vi "Main.vi"(11 "Module Admin":refnum<class "Delacor_lib_QMH_Module Admin.lvclass">) -> ()   [LabVIEW 2019, in "ContextHelp.lvlib"]
doc: "This template is based off of the Queued Message Handler design pattern and the Queued Message Handler project template that ships with LabVIEW.\n\nThe main difference is that the queue is private to this module and communication between modules is performed via Broadcast and Request events.\n\nRequest events are wrapped in public API methods and are handled in the Event Handling Loop (EHL) of this VI. Any module can register for Broadcast events sent by this module. The EHL generates messages based on user interface actions.\n\nThe Message Handling Loop (MHL) processes messages generated by the EHL, or by other messages. The messages are string values, so new messages can be added easily to the Message Cases case structure in the MHL. Each message cluster can also provide an optional value for Message Data, which is a variant that can be converted to whatever message-specific data is required.\n_____\nBased on DQMH Project Template 6.1.0.94.\n____\nPantherLAB Templates 1.0.0.5\nCopyright (c) 2022, PantherLAB"
uses:
  ContextHelp.lvlib
  <vilib>/Delacor/Delacor QMH/Libraries/Module Admin_class/Delacor_lib_QMH_Module Admin.lvclass
  Module Data--cluster.ctl
  <vilib>/Delacor/Delacor QMH/Libraries/Message Queue_class/Delacor_lib_QMH_Message Queue.lvclass/Delacor_lib_QMH_Message Queue.ctl
  Stop Argument--cluster.ctl
  <vilib>/Delacor/Delacor QMH/Libraries/Module Admin_class/Delacor_lib_QMH_Module Admin.lvclass/Delacor_lib_QMH_Module Admin.ctl
  Draw Panel Into Subpanel Argument--cluster.ctl
  Remove Panel from Subpanel Argument--cluster.ctl
  <vilib>/Delacor/Delacor QMH/Libraries/Message Queue_class/Delacor_lib_QMH_Enqueue Message (Single).vi
  <vilib>/Delacor/Delacor QMH/Libraries/Module Admin_class/Delacor_lib_QMH_Get External Launch.vi
  <vilib>/Utility/error.llb/Error Cluster From Error Code.vi
  <vilib>/ErrorRing/Error Ring.xnode
  <vilib>/Delacor/Delacor QMH/Libraries/Message Queue_class/Delacor_lib_QMH_Message Queue.lvclass
  Panther Dashboard/Panther Dashboard.lvlib
  Shared/Shared.lvlib
panel:
  out "Status":string
  out "error out":errorcluster
  in  "Edit Project Description":bool caption="Project Documentation"
  in  "Project Description":string
  in  "Edit Module Description":bool caption="Module Description"
  in  "Module Description":string
  in  "Edit VI":bool caption="Event Connector Pane- Edit"
  out "Event Connector Pane":picture
  in  "Event Description":string
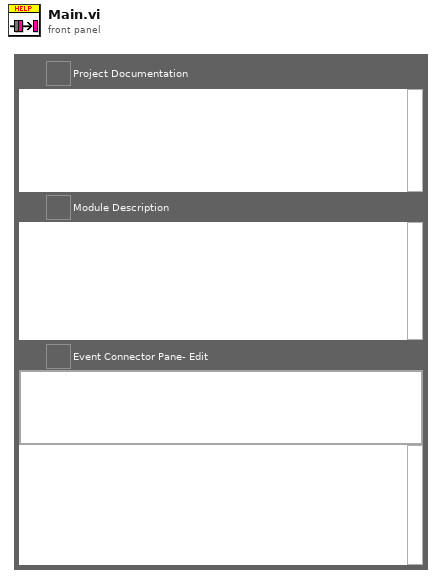
[diagram p1: front panel]
types:
  T1 = typedef "ContextHelp.lvlib/Request Events--cluster.ctl" = cluster{"Stop Module":refnum<user-event>, "Show Panel":refnum<user-event>, "Hide Panel":refnum<user-event>, "Get Module Execution Status":refnum<user-event>, "Show Diagram":refnum<user-event>, "Wake up Helper Loop":refnum<user-event>, "Put Helper Loop to Sleep":refnum<user-event>, "Draw Panel Into Subpanel":refnum<user-event>, "Remove Panel from Subpanel":refnum<user-event>, "Refresh Panther Dashboard Broadcasts":refnum<user-event>}
  T2 = typedef "Panther Dashboard.lvlib/Broadcast Events--cluster.ctl" = cluster{"Module Did Init":refnum<user-event>, "Status Updated":refnum<user-event>, "Error Reported":refnum<user-event>, "Module Did Stop":refnum<user-event>, "Update Module Execution Status":refnum<user-event>, "References Updated":refnum<user-event>, "Projects Updated":refnum<user-event>, "Targets Updated":refnum<user-event>, "Progress updated":refnum<user-event>, "Scale Updated":refnum<user-event>, "Connector Pane Updated":refnum<user-event>, "Documentation Updated":refnum<user-event>, "Module Type Updated":refnum<user-event>, "Theme Updated":refnum<user-event>, "Project Description Updated":refnum<user-event>}
  T3 = typedef "ContextHelp.lvlib/Module Data--cluster.ctl" = cluster{"Status":string, "SubPanel":refnum<vi>, "Panel Status":bool}
  T4 = enum8{"Enabled", "Disabled", "Disabled and Grayed Out"}
  T5 = enum32{"invalid lock state", "Not Locked", "Locked (No Password)", "Password-protected"}
  T6 = typedef "ContextHelp.lvlib/Stop Argument--cluster.ctl" = cluster{"Origin":string, "Exit via Stop Module Req?":bool, "Wait for Module to stop?":bool}
  T7 = typedef "ContextHelp.lvlib/Draw Panel Into Subpanel Argument--cluster.ctl" = cluster{"Sub Panel":refnum<vi>}
  T8 = typedef "ContextHelp.lvlib/Remove Panel from Subpanel Argument--cluster.ctl" = cluster{"Boolean":bool}
  T9 = enum32{"Invalid", "Standard", "Closed", "Hidden", "Minimized", "Maximized"}
  T10 = typedef "LVRectTypeDef.ctl" = cluster{"Left":i16, "Top":i16, "Right":i16, "Bottom":i16}
  T11 = typedef "Panther Dashboard.lvlib/Documentation--cluster.ctl" = cluster{"Module Description":string, "Event Description":string}
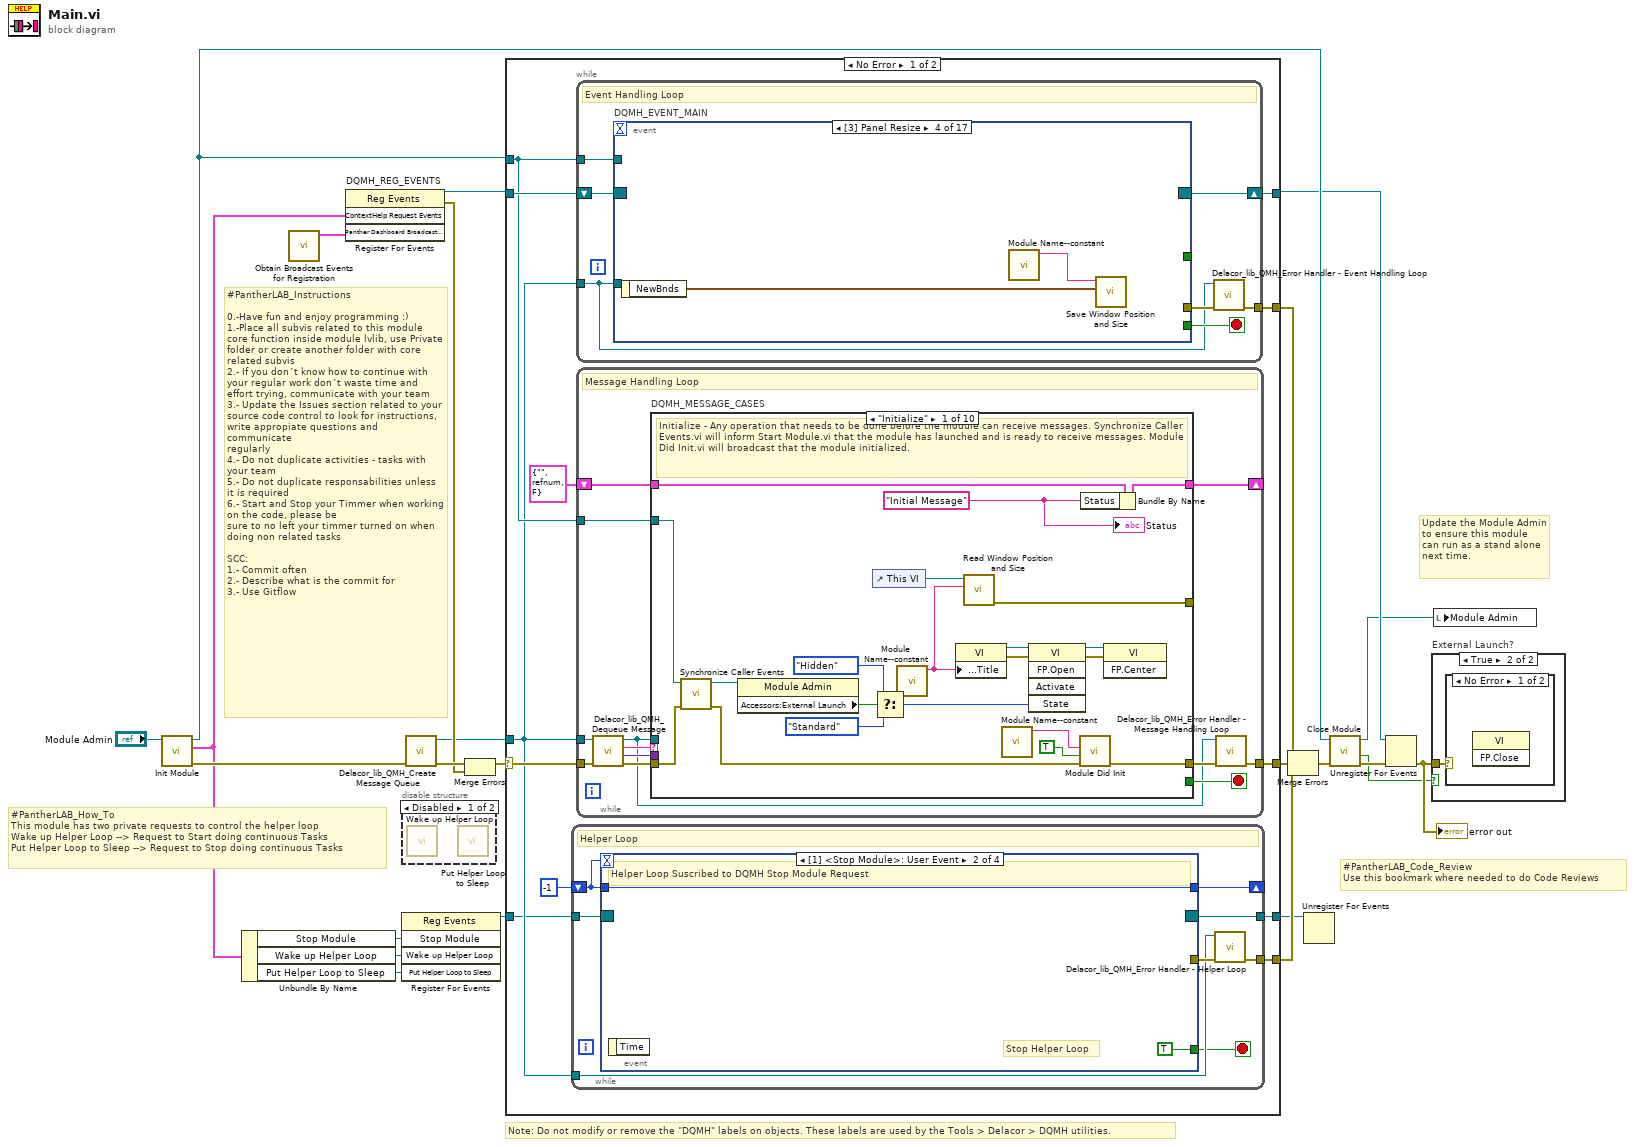
[diagram p0: block diagram]
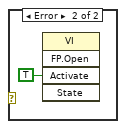
[diagram p4: hidden frame]
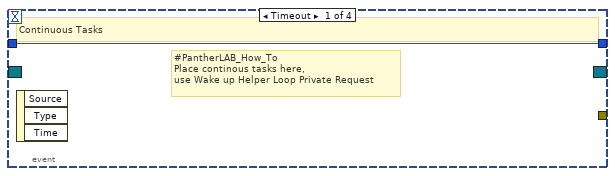
[diagram p5: hidden frame]
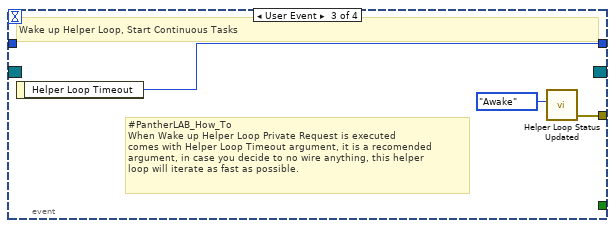
[diagram p6: hidden frame]
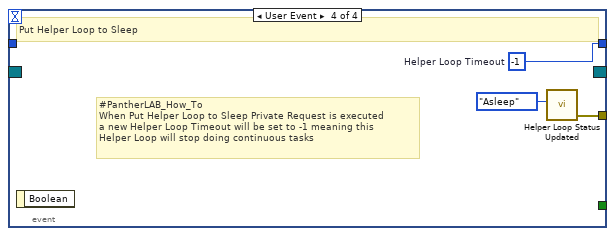
[diagram p7: hidden frame]
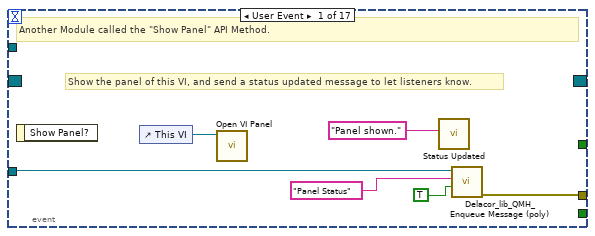
[diagram p8: hidden frame]
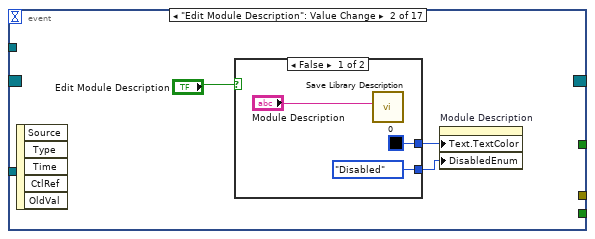
[diagram p9: hidden frame]
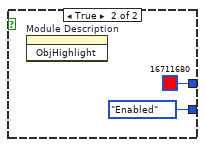
[diagram p10: hidden frame]
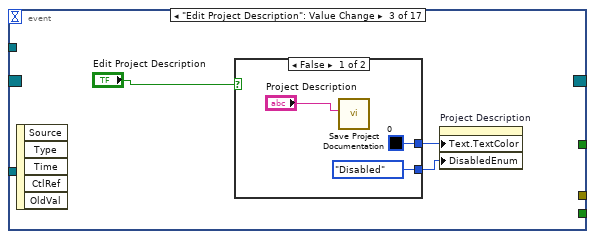
[diagram p11: hidden frame]
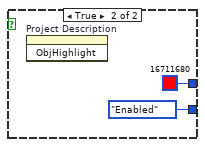
[diagram p12: hidden frame]
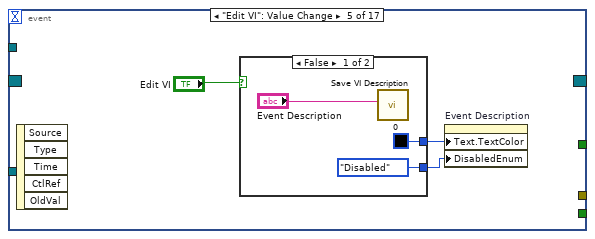
[diagram p13: hidden frame]
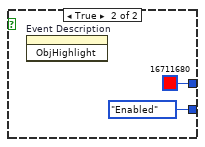
[diagram p14: hidden frame]
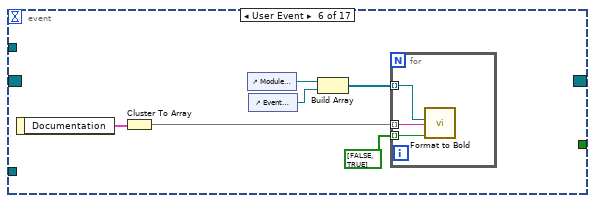
[diagram p15: hidden frame]
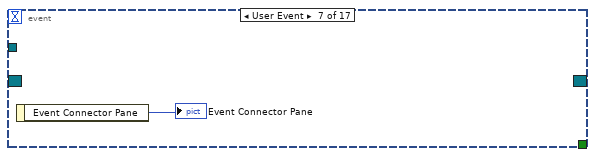
[diagram p16: hidden frame]
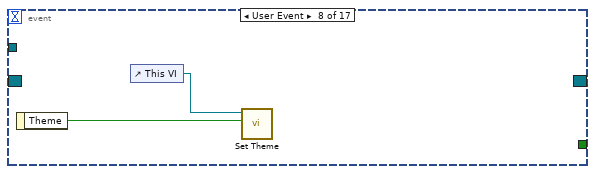
[diagram p17: hidden frame]
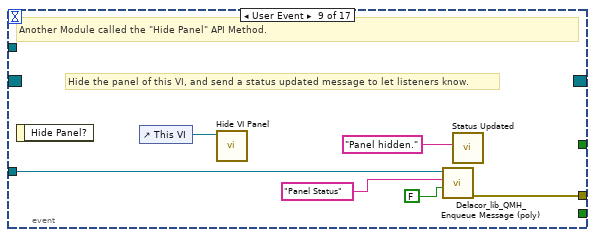
[diagram p18: hidden frame]
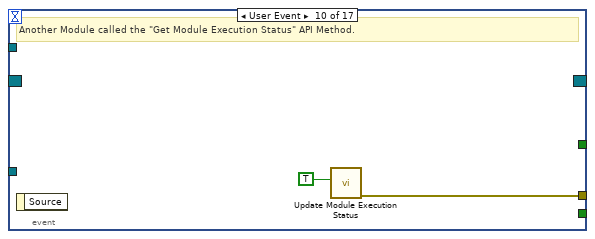
[diagram p19: hidden frame]
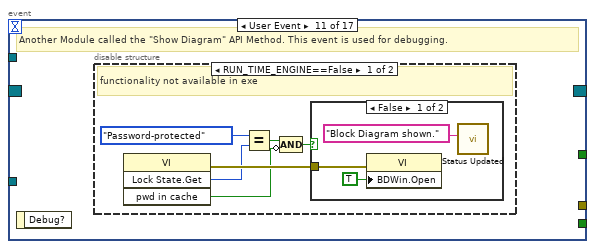
[diagram p20: hidden frame]
diagram:
  # "#PantherLAB_Instructions\n\n0.-Have fun and enjoy programming :)\n1.-Place all subvis related to this module core function inside module lvlib, use Private folder or create another folder with core related subvis \n2.- If you don´t know how to continue with your regular work don´t waste time and effort trying, communicate with your team\n3.- Update the Issues section related to your source code control to look for instructions, write appropiate questions and communicate\nregularly\n4.- Do not duplicate activities - tasks with your team\n5.- Do not duplicate responsabilities unless it is required\n6.- Start and Stop your Timmer when working on the code, please be\nsure to no left your timmer turned on when doing non related tasks\n\nSCC:\n1.- Commit often\n2.- Describe what is the commit for\n3.- Use Gitflow"
  # "#PantherLAB_Code_Review\nUse this bookmark where needed to do Code Reviews"
  # "#PantherLAB_How_To\nThis module has two private requests to control the helper loop\nWake up Helper Loop --> Request to Start doing continuous Tasks\nPut Helper Loop to Sleep --> Request to Stop doing continuous Tasks"
  # "Note: Do not modify or remove the \"DQMH\" labels on objects. These labels are used by the Tools > Delacor > DQMH utilities."
  # "Update the Module Admin to ensure this module can run as a stand alone next time."
  n1 = call "Init Module.vi"("Singleton Module Admin in"="Module Admin") -> ("error out"=w23:errorcluster, "ContextHelp Request Events"=w7:T1, "Singleton Module Admin out"=w14:refnum<class "Delacor_lib_QMH_Module Admin.lvclass">)  [unwired: 8 in]
  n2 = Unbundle By Name(w7) -> ("Stop Module"=w6:refnum<user-event>, "Wake up Helper Loop"=w3:refnum<user-event>, "Put Helper Loop to Sleep"=w2:refnum<user-event>)
  n3 = call "Obtain Broadcast Events for Registration.vi"() -> ("Panther Dashboard Broadcast Events"=w1:T2)  [unwired: 9 in, 2 out]
  n4 = register-events "DQMH_REG_EVENTS"(w7, w1) -> (reference out=w12:refnum<event-registration>, error out=w16:errorcluster)  [unwired: 2 in]
  n5 = register-events(w6, w3, w2) -> (reference out=w5:refnum<event-registration>)  [unwired: 2 in, 1 out]
  n6 = disable-structure shown="Disabled" {
    frame Disabled {
      n7 = call "Wake up Helper Loop.vi"() -> ()  [unwired: 11 in, 1 out]
      n8 = call "Put Helper Loop to Sleep.vi"() -> ()  [unwired: 11 in, 1 out]
    }
    frame Enabled {
    }
  }
  n9 = call <vilib>:"Delacor_lib_QMH_Create Message Queue.vi"("error in"=w23) -> ("error out"=w18:errorcluster, "Message Queue"=w11:refnum<class "Delacor_lib_QMH_Message Queue.lvclass">)  [unwired: 9 in]
  n10 = Merge Errors(w18, w16) -> (w17:errorcluster)
  n11 = case shown="No Error" w17 {
    selector: w17 -> [w34 w287]
    tunnel: [w36 w286] -> w24
    tunnel: [w32 w285] -> w13
    tunnel: w12 -> [w30 w285]
    tunnel: w11 -> [w28 w280]
    tunnel: [w35 _] -> w21
    tunnel: w14 -> [w29 w281]
    tunnel: w5 -> [w27 w279]
    tunnel: [w25 w279] -> w4
    tunnel: [w33 _] -> w15
    frame No Error {
      n12 = while {
        tunnel: w28 -> [w38]
        tunnel: w27 -> [w42]
        shift-right: [w40] -> _
        shift-left: -1 -> [w41]
        tunnel: [w39] -> w25
        tunnel: [w44] -> w33
        stop <- w37 stop-if-true
        # "Helper Loop"
        n13 = event shown="[1] <Stop Module>: User Event" {
          selector: w42 -> [_ _ _ _]
          dyn-events: [_ _ _ _] -> w39
          timeout: w41 -> [_ _ _ _]
          tunnel: w41 -> [w45 w47 _ _]
          tunnel: [w45 w47 w49 w51] -> w40
          tunnel: [_ TRUE _ _] -> w37
          tunnel: [_ _ w50 w53] -> w43
          event Timeout {
            # "#PantherLAB_How_To\nPlace continous tasks here,\nuse Wake up Helper Loop Private Request"
            # "Continuous Tasks"
            n14 = event-data() -> ()  [unwired: 1 in, 3 out]
          }
          event User Event {
            # "Stop Helper Loop"
            # "Helper Loop Suscribed to DQMH Stop Module Request"
            n15 = event-data() -> ()  [unwired: 1 in, 1 out]
          }
          event User Event {
            # "#PantherLAB_How_To\nWhen Wake up Helper Loop Private Request is executed\ncomes with Helper Loop Timeout argument, it is a recomended\nargument, in case you decide to no wire anything, this helper\nloop will iterate as fast as possible."
            # "Wake up Helper Loop, Start Continuous Tasks"
            n16 = event-data() -> ("Helper Loop Timeout"=w49:i32)  [unwired: 1 in]
            n17 = call "Helper Loop Status Updated.vi"("Helper Loop Status"=enum16{"Awake", "Asleep"}."Awake") -> ("error out"=w50:errorcluster)  [unwired: 10 in]
          }
          event User Event {
            w51 = -1  # Helper Loop Timeout
            # "#PantherLAB_How_To\nWhen Put Helper Loop to Sleep Private Request is executed\na new Helper Loop Timeout will be set to -1 meaning this\nHelper Loop will stop doing continuous tasks"
            # "Put Helper Loop to Sleep"
            n18 = event-data() -> ()  [unwired: 1 in, 1 out]
            n19 = call "Helper Loop Status Updated.vi"("Helper Loop Status"=enum16{"Awake", "Asleep"}."Asleep") -> ("error out"=w53:errorcluster)  [unwired: 10 in]
          }
        }
        n20 = call-dynamic "Delacor_lib_QMH_Error Handler - Helper Loop.vi"("error in"=w43, "Message Queue in"=w38) -> ("dup error in"=w44:errorcluster)  [unwired: 8 in, 1 out]
      }
      n21 = while {
        tunnel: w28 -> [w54]
        shift-right: [w57] -> w32
        shift-left: w30 -> [w58]
        tunnel: [w59] -> w35
        tunnel: w29 -> [w55]
        stop <- w56 stop-if-true
        # "Event Handling Loop"
        n22 = event "DQMH_EVENT_MAIN" shown="[3] Panel Resize" {
          selector: w58 -> [_ _ _ _ _ _ _ _ _ _ _ _ _ _ _ w159 _]
          dyn-events: [_ _ _ _ _ _ _ _ _ _ _ _ _ _ _ w158 _] -> w57
          timeout: _ -> [_ _ _ _ _ _ _ _ _ _ _ _ _ _ _ _ _]
          tunnel: [_ _ _ _ _ _ _ _ _ _ _ TRUE ("Discard?") _ _ _ _ _] -> w56
          tunnel: w54 -> [w63 _ _ _ _ _ _ _ w105 _ _ w129 w136 w148 w154 _ _]
          tunnel: [w66 _ _ _ _ _ _ _ w110 w112 _ w132 w138 w149 w155 _ _] -> w60
          tunnel: w55 -> [_ _ _ _ _ _ _ _ _ _ _ _ w135 _ _ _ _]
          tunnel: [_ _ _ _ _ _ _ _ _ _ _ _ _ _ _ w156 _] -> _
          event User Event {
            # "Show the panel of this VI, and send a status updated message to let listeners know."
            # "Another Module called the \"Show Panel\" API Method."
            n23 = event-data() -> ()  [unwired: 1 in, 1 out]
            n24 = control-ref of="This VI"() -> (w65:refnum<vi>)
            n25 = call "Open VI Panel.vi"("VI"=w65) -> ()  [unwired: 10 in, 1 out]
            n26 = call "Status Updated.vi"("Status"="Panel shown." ("format string")) -> ()  [unwired: 10 in, 1 out]
            n27 = call-poly <vilib>:"Delacor_lib_QMH_Enqueue Message (poly).vi"("Message Data"=TRUE, "Message"="Panel Status" ("format string"), "Message Queue in"=w63) -> ("error out"=w66:errorcluster)  [unwired: 7 in, 1 out]
          }
          event "Edit Module Description": Value Change {
            n28 = event-data() -> ()  [unwired: 1 in, 5 out]
            n29 = case shown="False" "Edit Module Description" {
              tunnel: [u32 0 u32 16711680] -> w68
              tunnel: [T4."Disabled" ("Disabled") T4."Enabled" ("Disabled")] -> w69
              frame False {
                n30 = call "Save Library Description.vi"("Library Description"="Module Description") -> ()  [unwired: 10 in, 1 out]
              }
              frame True {
                n31 = invoke on="Module Description" class="Str" method="ObjHighlight"() -> ()  [unwired: 3 in, 3 out]
              }
            }
            n32 = property on="Module Description" class="Str"("Text.TextColor"=w68, "DisabledEnum"=w69) -> ()  [unwired: 2 in, 2 out]
          }
          event "Edit Project Description": Value Change {
            n33 = event-data() -> ()  [unwired: 1 in, 5 out]
            n34 = case shown="False" "Edit Project Description" {
              tunnel: [u32 0 u32 16711680] -> w76
              tunnel: [T4."Disabled" ("Disabled") T4."Enabled" ("Disabled")] -> w77
              frame False {
                n35 = call "Save Project Documentation.vi"("Project Description"="Project Description") -> ()  [unwired: 10 in, 1 out]
              }
              frame True {
                n36 = invoke on="Project Description" class="Str" method="ObjHighlight"() -> ()  [unwired: 3 in, 3 out]
              }
            }
            n37 = property on="Project Description" class="Str"("Text.TextColor"=w76, "DisabledEnum"=w77) -> ()  [unwired: 2 in, 2 out]
          }
          event Panel Resize {
            n38 = event-data() -> ("NewBnds"=w84:T10)  [unwired: 1 in]
            n39 = call "Module Name--constant.vi"() -> ("Module Name"=w83:string)  [unwired: 11 in]
            n40 = call "Save Window Position and Size.vi"("NewBnds"=w84, "Position Key"=w83) -> ()  [unwired: 9 in, 1 out]
          }
          event "Edit VI": Value Change {
            n41 = event-data() -> ()  [unwired: 1 in, 5 out]
            n42 = case shown="False" "Edit VI" {
              tunnel: [u32 0 u32 16711680] -> w86
              tunnel: [T4."Disabled" ("Disabled") T4."Enabled" ("Disabled")] -> w87
              frame False {
                n43 = call "Save VI Description.vi"("VI Description"="Event Description") -> ()  [unwired: 10 in, 1 out]
              }
              frame True {
                n44 = invoke on="Event Description" class="Str" method="ObjHighlight"() -> ()  [unwired: 3 in, 3 out]
              }
            }
            n45 = property on="Event Description" class="Str"("Text.TextColor"=w86, "DisabledEnum"=w87) -> ()  [unwired: 2 in, 2 out]
          }
          event User Event {
            n46 = event-data() -> ("Documentation"=w98:T11)  [unwired: 1 in]
            n47 = Cluster To Array(cluster=w98) -> (array=w96:string[])
            n48 = control-ref of="Module Description"() -> (w94:refnum<vi>)
            n49 = control-ref of="Event Description"() -> (w93:refnum<vi>)
            n50 = Build Array(w94, w93) -> (w95:refnum<vi>[])
            n51 = for {
              tunnel: bool[] [FALSE, TRUE] ("Adjust Height?") -> [w101] mode=indexing
              tunnel: w96 -> [w100] mode=indexing
              tunnel: w95 -> [w99] mode=indexing
              n52 = call "Format to Bold.vi"("Adjust Height?"=w101, "String Value"=w100, "String Ref"=w99) -> ()  [unwired: 9 in]
            }
          }
          event User Event {
            n53 = event-data() -> ("Event Connector Pane"=→"Event Connector Pane":picture)  [unwired: 1 in]
          }
          event User Event {
            n54 = event-data() -> ("Theme"=w103:bool)  [unwired: 1 in]
            n55 = control-ref of="This VI"() -> (w104:refnum<vi>)
            n56 = call "Set Theme.vi"("Dark?"=w103, "VI in"=w104) -> ()  [unwired: 10 in]
          }
          event User Event {
            # "Hide the panel of this VI, and send a status updated message to let listeners know."
            # "Another Module called the \"Hide Panel\" API Method."
            n57 = event-data() -> ()  [unwired: 1 in, 1 out]
            n58 = control-ref of="This VI"() -> (w109:refnum<vi>)
            n59 = call "Hide VI Panel.vi"("VI"=w109) -> ()  [unwired: 10 in, 1 out]
            n60 = call-poly <vilib>:"Delacor_lib_QMH_Enqueue Message (poly).vi"("Message Data"=FALSE, "Message"="Panel Status" ("format string"), "Message Queue in"=w105) -> ("error out"=w110:errorcluster)  [unwired: 7 in, 1 out]
            n61 = call "Status Updated.vi"("Status"="Panel hidden." ("format string")) -> ()  [unwired: 10 in, 1 out]
          }
          event User Event {
            # "Another Module called the \"Get Module Execution Status\" API Method."
            n62 = event-data() -> ()  [unwired: 1 in, 1 out]
            n63 = call "Update Module Execution Status.vi"("Running?"=TRUE) -> ("error out"=w112:errorcluster)  [unwired: 10 in]
          }
          event User Event {
            # "Another Module called the \"Show Diagram\" API Method. This event is used for debugging."
            n64 = event-data() -> ()  [unwired: 1 in, 1 out]
            n65 = disable-structure shown="RUN_TIME_ENGINE==False" {
              frame condition #0 (active) {
                # "functionality not available in exe"
                n66 = invoke class="VI" method="Lock State.Get"() -> (error out=w118:errorcluster, "Get Lock State"=w117:T5, "pwd in cache"=w114:bool)  [unwired: 4 in, 1 out]
                n67 = Equal?(x=T5."Password-protected", y=w117) -> (x = y?=w115:bool)
                n68 = Compound Arithmetic op=AND(w115, invert w114) -> (w113:bool)
                n69 = case shown="False" w113 {
                  tunnel: w118 -> [w121 _]
                  frame False {
                    n70 = property class="VI"(error in=w121, "BDWin.Open"=TRUE ("Block Diagram Window:Open")) -> ()  [unwired: 1 in, 2 out]
                    n71 = call "Status Updated.vi"("Status"="Block Diagram shown." ("format string")) -> ()  [unwired: 10 in, 1 out]
                  }
                  frame True {
                    # "Password-protected VI, and the password is not in the cache. Do not show the diagram."
                  }
                }
              }
              frame condition #1 {
              }
            }
          }
          event User Event {
            # "The Stop Module Event can get fired from the Exit message in the MHL. The queue gets destroyed in that case. If the queue no longer exists, the Enqueue Exit as a priority message will return error 1. It is safe to ignore, because the module is already exiting."
            # "Another Module called the \"Stop Module\" API Method  or the Message Handling Loop below."
            n72 = event-data() -> ("Origin"=w128:string, "Exit via Stop Module Req?"=w124:bool, "Wait for Module to stop?"=w123:bool)  [unwired: 1 in]
            n73 = local write "Status"(w128) -> ()
            n74 = Bundle By Name(cluster=T6 {"Origin"="", "Exit via Stop Module Req?"=FALSE, "Wait for Module to stop?"=FALSE} ("Stop Argument"), "Exit via Stop Module Req?"=w124, "Wait for Module to stop?"=w123) -> (w122:T6)
            n75 = call-poly <vilib>:"Delacor_lib_QMH_Enqueue Message (poly).vi"("Priority Message? (F)"=TRUE, "Message Data"=w122, "Message"="Exit", "Message Queue in"=w129) -> ("error out"=w133:errorcluster)  [unwired: 6 in, 1 out]
            n76 = call <vilib>:"Clear Errors.vi"("error in (no error)"=w133, "specific error code to clear (0: all)"=1) -> ("error out"=w132:errorcluster)  [unwired: 4 in, 1 out]
          }
          event Panel Close? {
            w137 = TRUE  # Discard the event, the MHL is responsible for closing and stopping this VI.
            # "Hide the panel or send the 'Exit' message if the user clicks the 'X' on the module main VI panel."
            n77 = event-data() -> ()  [unwired: 1 in, 1 out]
            n78 = property class="Module Admin"(reference=w135) -> ("Accessors:External Launch"=w134:bool)  [unwired: 1 in, 2 out]
            n79 = case shown="False" w134 {
              tunnel: w136 -> [_ w142]
              tunnel: [_ w143] -> w138
              frame True {
                # "If externally launched, clicking the 'X' hides the panel, but doesn't close it."
                n80 = control-ref of="This VI"() -> (w139:refnum<vi>)
                n81 = call "Hide VI Panel.vi"("VI"=w139) -> ()  [unwired: 10 in, 1 out]
              }
              frame False {
                # "If run as a stand-alone VI, clicking the panel 'X' stops the VI."
                n82 = call-poly <vilib>:"Delacor_lib_QMH_Enqueue Message (poly).vi"("Priority Message? (F)"=TRUE, "Message"="Exit", "Message Queue in"=w142) -> ("error out"=w143:errorcluster)  [unwired: 7 in, 1 out]
              }
            }
            n83 = event-data("Discard?"=w137) -> ()  [unwired: 1 in, 1 out]
          }
          event User Event {
            # "Another Module called the \"Draw your Panel into Subpanel\" API Method."
            n84 = event-data() -> ("Sub Panel"=w144:refnum<vi>)  [unwired: 1 in]
            n85 = Bundle(cluster=T7 {"Sub Panel"=refnum} ("Draw your Panel into Subpanel Argument"), "Sub Panel"=w144) -> (w145:T7)
            n86 = call-poly <vilib>:"Delacor_lib_QMH_Enqueue Message (poly).vi"("Message Data"=w145, "Message"="Draw Panel into Subpanel", "Message Queue in"=w148) -> ("error out"=w149:errorcluster)  [unwired: 7 in, 1 out]
          }
          event User Event {
            # "Another Module called the \"Remove Panel from Subpanel\" API Method."
            n87 = event-data() -> ("Boolean"=w150:bool)  [unwired: 1 in]
            n88 = Bundle(cluster=T8 {"Boolean"=FALSE} ("Remove Panel from Subpanel Argument"), "Boolean"=w150) -> (w151:T8)
            n89 = call-poly <vilib>:"Delacor_lib_QMH_Enqueue Message (poly).vi"("Message Data"=w151, "Message"="Remove Panel from Subpanel", "Message Queue in"=w154) -> ("error out"=w155:errorcluster)  [unwired: 7 in, 1 out]
          }
          event User Event {
            # "Another Module called the \"Refresh Panther Dashboard Broadcasts\" API Method."
            n90 = event-data() -> ()  [unwired: 1 in, 1 out]
            n91 = call "Obtain Broadcast Events for Registration.vi"() -> ("Already running?"=w156:bool, "Panther Dashboard Broadcast Events"=w157:T2)  [unwired: 9 in, 1 out]
            n92 = register-events "Refresh Panther Broadcasts"(reference=w159, w157) -> (reference out=w158:refnum<event-registration>)  [unwired: 2 in, 1 out]
          }
          event User Event {
            n93 = event-data() -> ("Project Description"=w160:string)  [unwired: 1 in]
            n94 = local write "Project Description"(w160) -> ()
          }
        }
        n95 = call-dynamic "Delacor_lib_QMH_Error Handler - Event Handling Loop.vi"("error in"=w60, "Message Queue in"=w54) -> ("dup error in"=w59:errorcluster)  [unwired: 8 in, 1 out]
      }
      n96 = while {
        tunnel: w28 -> [w163]
        shift-right: [w167] -> _
        shift-left: T3 {"Status"="", "SubPanel"=refnum, "Panel Status"=FALSE} ("Data Cluster") -> [w168]
        tunnel: w34 -> [w171]
        tunnel: [w169] -> w36
        tunnel: w29 -> [w161]
        stop <- w166 stop-if-true
        # "Message Handling Loop"
        n97 = call-dynamic "Delacor_lib_QMH_Dequeue Message.vi"("error in"=w171, "Message Queue in"=w163) -> ("error out"=w170:errorcluster, "Message Data"=w164:variant, "Message"=w165:string, "Message Queue out"=w162:refnum<class "Delacor_lib_QMH_Message Queue.lvclass">)  [unwired: 6 in]
        n98 = case "DQMH_MESSAGE_CASES" shown="\"Initialize\"" w165 {
          selector: w165 -> [_ _ _ _ _ _ _ _ _ w266]
          tunnel: w162 -> [_ _ _ _ _ _ _ w232 w258 _]
          tunnel: w170 -> [w191 w195 w206 w215 w224 w227 w229 w239 w264 w268]
          tunnel: [w189 w195 w204 w214 w223 w226 w229 w235 w261 w269] -> w172
          tunnel: w168 -> [w181 w194 w203 w210 w222 w225 w228 w234 w250 w267]
          tunnel: [w180 w194 w197 w210 w219 w225 w228 w234 w250 w267] -> w167
          tunnel: [_ _ _ _ _ _ _ _ w257 _] -> w166
          tunnel: w164 -> [_ _ w202 w212 w221 _ _ w233 w256 _]
          tunnel: w161 -> [w182 _ _ _ _ _ _ w231 w251 _]
          tunnel: [w173 _ _ _ _ _ _ _ _ _] -> _
          frame "Initialize" {
            w176 = "Initial Message" ("Initial Message")
            # "Initialize - Any operation that needs to be done before the module can receive messages. Synchronize Caller Events.vi will inform Start Module.vi that the module has launched and is ready to receive messages. Module Did Init.vi will broadcast that the module initialized."
            n99 = call "Synchronize Caller Events.vi"("error in (no error)"=w191, "Singleton Module Admin in"=w182) -> ("error out"=w190:errorcluster, "Singleton Module Admin out"=w177:refnum<class "Delacor_lib_QMH_Module Admin.lvclass">)  [unwired: 8 in]
            n100 = property class="Module Admin"(reference=w177) -> ("Accessors:External Launch"=w186:bool)  [unwired: 1 in, 2 out]
            n101 = control-ref of="This VI"() -> (w175:refnum<vi>)
            n102 = Select(t=T9."Hidden" ("State"), s=w186, f=T9."Standard" ("State")) -> (s? t:f=w183:T9)
            n103 = call "Module Name--constant.vi"() -> ("Module Name"=w174:string)  [unwired: 11 in]
            n104 = property class="VI"("Front Panel.Title"=w174) -> (reference out=w188:refnum<vi>, error out=w193:errorcluster)  [unwired: 2 in]
            n105 = call "Read Window Position and Size.vi"("Position Key"=w174, "VI Refnum"=w175) -> ("error out"=w173:errorcluster)  [unwired: 9 in]
            n106 = call "Module Name--constant.vi"() -> ("Module Name"=w178:string)  [unwired: 11 in]
            n107 = invoke class="VI" method="FP.Open"(reference=w188, error in=w193, "State"=w183) -> (reference out=w187:refnum<vi>, error out=w192:errorcluster)  [unwired: 2 in, 3 out]
            n108 = call "Module Did Init.vi"("error in (no error)"=w190, "Initialized?"=TRUE, "Origin"=w178) -> ("error out"=w189:errorcluster)  [unwired: 8 in]
            n109 = Bundle By Name(cluster=w181, "Status"=w176) -> (w180:T3)
            n110 = invoke class="VI" method="FP.Center"(reference=w187, error in=w192) -> ()  [unwired: 1 in, 3 out]
            "Status" <- w176
          }
          frame "---Module Specific---" {
            # "Separator -- The following cases handle messages specific to this Module."
          }
          frame "Draw Panel into Subpanel" {
            # "#PantherLAB_How_To\nThis module request allows to draw Main.vi into any \nsubpanel provided"
            # "Request made to the module to draw itself into a subpanel provided"
            n111 = Variant To Data(error in=w206, type=T7 {"Sub Panel"=refnum} ("Draw your Panel into Subpanel Argument"), Variant=w202) -> (data=w200:T7, error out=w205:errorcluster)
            n112 = Unbundle By Name(w200) -> ("Sub Panel"=w198:refnum<vi>)
            n113 = control-ref of="This VI"() -> (w199:refnum<vi>)
            n114 = call "Draw Panel Into Subpanel Procedure.vi"("error in"=w205, "SubPanel in"=w198, "This VI"=w199) -> ("error out"=w204:errorcluster, "SubPanel out"=w196:refnum<vi>)  [unwired: 7 in]
            n115 = Bundle By Name(cluster=w203, "SubPanel"=w196) -> (w197:T3)
          }
          frame "Remove Panel from Subpanel" {
            # "Request to the module to remove itself from the subpanel"
            n116 = Variant To Data(error in=w215, type=T8 {"Boolean"=FALSE} ("Remove Panel from Subpanel Argument"), Variant=w212) -> (error out=w214:errorcluster)  [unwired: 1 out]
            n117 = Unbundle By Name(w210) -> ("Panel Status"=w208:bool, "SubPanel"=w209:refnum<vi>)
            n118 = invoke class="SubPnl" method="Remove VI"(reference=w209) -> (error out=w213:errorcluster)  [unwired: 2 in, 2 out]
            n119 = control-ref of="This VI"() -> (w207:refnum<vi>)
            n120 = case shown="True" w208 {
              tunnel: w213 -> [_ _]
              tunnel: w207 -> [w216 w217]
              frame False {
                # "Hiden"
                n121 = call "Hide VI Panel.vi"("VI"=w216) -> ()  [unwired: 10 in, 1 out]
              }
              frame True {
                # "Visible"
                n122 = call "Open VI Panel.vi"("VI"=w217) -> ()  [unwired: 10 in, 1 out]
              }
            }
          }
          frame "Panel Status" {
            n123 = Variant To Data(error in=w224, type=TRUE, Variant=w221) -> (data=w218:bool, error out=w223:errorcluster)
            n124 = Bundle By Name(cluster=w222, "Panel Status"=w218) -> (w219:T3)
          }
          frame "---Copy This Frame---" {
            # "Duplicate this frame when creating new messages.  Change this comment in the duplicated frame to describe this message."
            n125 = Merge Errors(w227) -> (w226:errorcluster)
          }
          frame "---Exit and Error Handling---" {
            # "Separator - The following cases handle errors and exit messages."
          }
          frame "Error" {
            # "#CodeRecommended - If you ever change the name of this \"Error\" message, you'll need to update the name in the Check Loop Error.vi as well."
            # "#CodeRecommended - If the module is running in standalone mode (External Launch = FALSE), this code will pop up an error dialog and call the 'Exit' message if an error occurs. Add more fine-grained error handling here."
            # "Error - Check the error message data and respond accordingly. This message is sent by the \"Error Handler\" VIs at the end of each loop in this application."
            n126 = property class="Module Admin"(reference=w231) -> ("Accessors:External Launch"=w230:bool)  [unwired: 1 in, 2 out]
            n127 = Variant To Data(error in=w239, type=errorcluster {"status"=FALSE, "code"=0, "source"=""} ("error constant"), Variant=w233) -> (data=w240:errorcluster, error out=w237:errorcluster)
            n128 = call "Error Reported.vi"("Error"=w240) -> ()  [unwired: 10 in, 1 out]
            n129 = case shown="False" w230 {
              tunnel: [w245 _] -> w236
              tunnel: w232 -> [w243 _]
              tunnel: w240 -> [w244 _]
              frame False {
                # "If the module is running standalone, then pop up an error dialog and call the \"Exit\" message."
                n130 = call <vilib>:"Simple Error Handler.vi"("error in (no error)"=w244) -> ()  [unwired: 4 in, 5 out]
                n131 = call-poly <vilib>:"Delacor_lib_QMH_Enqueue Message (poly).vi"("Priority Message? (F)"=TRUE, "Message"="Exit", "Message Queue in"=w243) -> ("error out"=w245:errorcluster)  [unwired: 7 in, 1 out]
              }
              frame True {
                # "If the module was launched externally, calling the Error Reported broadcast VI is the only action performed by the \"Error\" message. The module's caller can then process the error appropriately."
              }
            }
            n132 = Merge Errors(w237, w236) -> (w235:errorcluster)
            n133 = local write "error out"(w235) -> ()
          }
          frame "Exit" {
            w255 = 91  # 91: not all Exit messages will have an argument
            w257 = TRUE  # Stop the VI
            # "Release the message queue reference"
            # "Exit - Exit the application."
            n134 = Variant To Data(error in=w264, type=T6 {"Origin"="", "Exit via Stop Module Req?"=FALSE, "Wait for Module to stop?"=FALSE} ("Stop Argument"), Variant=w256) -> (data=w253:T6, error out=w260:errorcluster)
            n135 = call <vilib>:"Clear Errors.vi"("error in (no error)"=w260, "specific error code to clear (0: all)"=w255) -> ("error out"=w263:errorcluster)  [unwired: 4 in, 1 out]
            n136 = Unbundle By Name(w250) -> ("SubPanel"=w249:refnum<vi>)
            n137 = control-ref of="This VI"() -> (w252:refnum<vi>)
            n138 = invoke class="SubPnl" method="Remove VI"(reference=w249) -> ()  [unwired: 2 in, 3 out]
            n139 = control-ref of="This VI"() -> (w248:refnum<vi>)
            n140 = call-dynamic "Delacor_lib_QMH_Release Message Queue.vi"("error in"=w263, "Message Queue"=w258) -> ("error out"=w262:errorcluster)  [unwired: 9 in]
            n141 = call "Handle Exit.vi"("Stop Argument"=w253, "Admin in"=w251, "VI reference"=w252) -> ("error out"=w259:errorcluster)  [unwired: 7 in, 1 out]
            n142 = property class="VI"(reference=w248) -> ("Front Panel.PanelBounds"=w247:T10)  [unwired: 1 in, 2 out]
            n143 = Merge Errors(w262, w259) -> (w261:errorcluster)
            n144 = call "Module Name--constant.vi"() -> ("Module Name"=w246:string)  [unwired: 11 in]
            n145 = call "Save Window Position and Size.vi"("NewBnds"=w247, "Position Key"=w246) -> ()  [unwired: 9 in, 1 out]
          }
          frame Default {
            # "'Default' case only runs if there is a message that isn't defined in any of the other cases.  Output a programming error."
            n146 = call "Module Name--constant.vi"() -> ("Module Name"=w265:string)  [unwired: 11 in]
            n147 = xnode "Error Ring"("parameter 0"=w266, "parameter 1"=w265) -> ("error out"=w270:errorcluster)
            n148 = Merge Errors(w268, w270) -> (w269:errorcluster)
          }
        }
        n149 = call-dynamic "Delacor_lib_QMH_Error Handler - Message Handling Loop.vi"("error in"=w172, "Message Queue in"=w162) -> ("dup error in"=w169:errorcluster)  [unwired: 8 in, 1 out]
      }
    }
    frame Error {
      # "Synchronize Caller Events.vi will inform Start Module.vi that the module has launched and will let the code calling Start Module.vi register for broadcasts and would permit the caller receive the broadcast that an error occurred at launch time."
      n150 = call-dynamic "Delacor_lib_QMH_Release Message Queue.vi"("error in"=w287, "Message Queue"=w280) -> ("error out"=w286:errorcluster)  [unwired: 9 in]
      n151 = call "Synchronize Caller Events.vi"("Singleton Module Admin in"=w281) -> ("error out"=w288:errorcluster)  [unwired: 9 in, 1 out]
      n152 = call "Module Name--constant.vi"() -> ("Module Name"=w284:string)  [unwired: 11 in]
      n153 = Format Into String(format string="An error occurred during initialization. %s is no longer running.", w284) -> (resulting string=w282:string)  [unwired: 2 in, 1 out]
      n154 = Merge Errors(w286, w288) -> (w289:errorcluster)
      n155 = call "Error Reported.vi"("Additional Information"=w282, "Error"=w289) -> ()  [unwired: 9 in, 1 out]
    }
  }
  n156 = Merge Errors(w21, w24, w15) -> (w20:errorcluster)
  n157 = Unregister For Events(event registration refnum=w4) -> ()  [unwired: 1 in, 1 out]
  n158 = call "Close Module.vi"("error in (no error)"=w20, "Module Admin in"=w14) -> ("error out"=w22:errorcluster, "External Launch"=w8:bool, "Module Admin out"=w9:refnum<class "Delacor_lib_QMH_Module Admin.lvclass">)  [unwired: 7 in]
  n159 = Unregister For Events(event registration refnum=w13, error in=w22) -> (error out=w19:errorcluster)
  "error out" <- w19
  n160 = case "External Launch?" shown="True" w8 {
    tunnel: w19 -> [_ w290]
    frame False {
    }
    frame True {
      n161 = case shown="No Error" w290 {
        frame No Error {
          n162 = invoke class="VI" method="FP.Close"() -> ()  [unwired: 3 in, 3 out]
        }
        frame Error {
          n163 = invoke class="VI" method="FP.Open"("Activate"=TRUE ("Activate?")) -> ()  [unwired: 4 in, 5 out]
        }
      }
    }
  }
  n164 = local write "Module Admin"(w9) -> ()
